vi "PH_Calorimeter_USB.contents.vi"   [LabVIEW 2014, in "PH_Calorimeter_USB.lvlib"]
doc: "This class is forseen to get the data and to calculate the energy of the calorimeter which are taken by the use of a NI USB-6009 I/O device.\nThis class is part of the PHELIX user layer."
uses:
  PH_Calorimeter_USB.lvlib
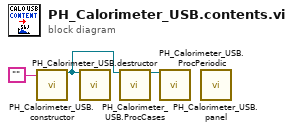
[diagram p0: block diagram]
diagram:
  n1 = call "PH_Calorimeter_USB.constructor.vi"("name"="") -> ("i ref out"=w1:refnum<vi>)  [unwired: 16 in, 2 out]
  n2 = call "PH_Calorimeter_USB.destructor.vi"("i ref in"=w1) -> ()  [unwired: 18 in, 1 out]
  n3 = call "PH_Calorimeter_USB.ProcCases.vi"("i ref in"=w1) -> ("i ref out"=w3:refnum<vi>)  [unwired: 16 in, 2 out]
  n4 = call "PH_Calorimeter_USB.ProcPeriodic.vi"("i ref in"=w3) -> ()  [unwired: 16 in, 3 out]
  n5 = call "PH_Calorimeter_USB.panel.vi"() -> ()  [unwired: 19 in, 1 out]
